vi "Get Measurement Plug-in API Paths.vi"(11 "error in":errorcluster) -> (6 "meas plugin api paths":path[](array[path]), 15 "error out":errorcluster)   [LabVIEW 2021, in "Path Functions.lvlib"]
uses:
  Path Functions.lvlib
  e97babff-5d82-41c0-a956-71097acbec5b.vi
  Converter Reusables/Converter Reusables.lvlib
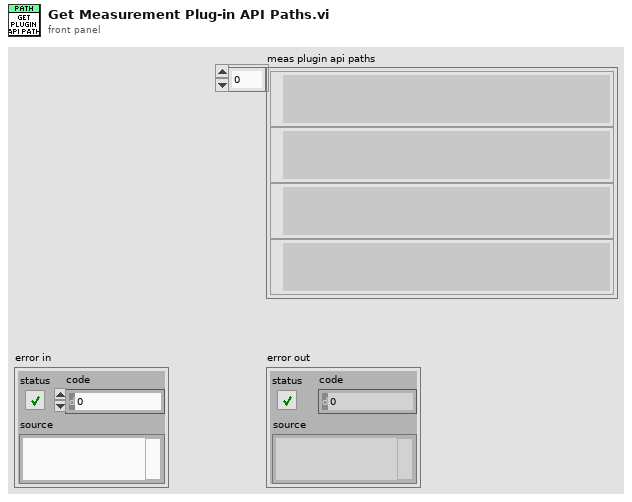
[diagram p1: front panel]
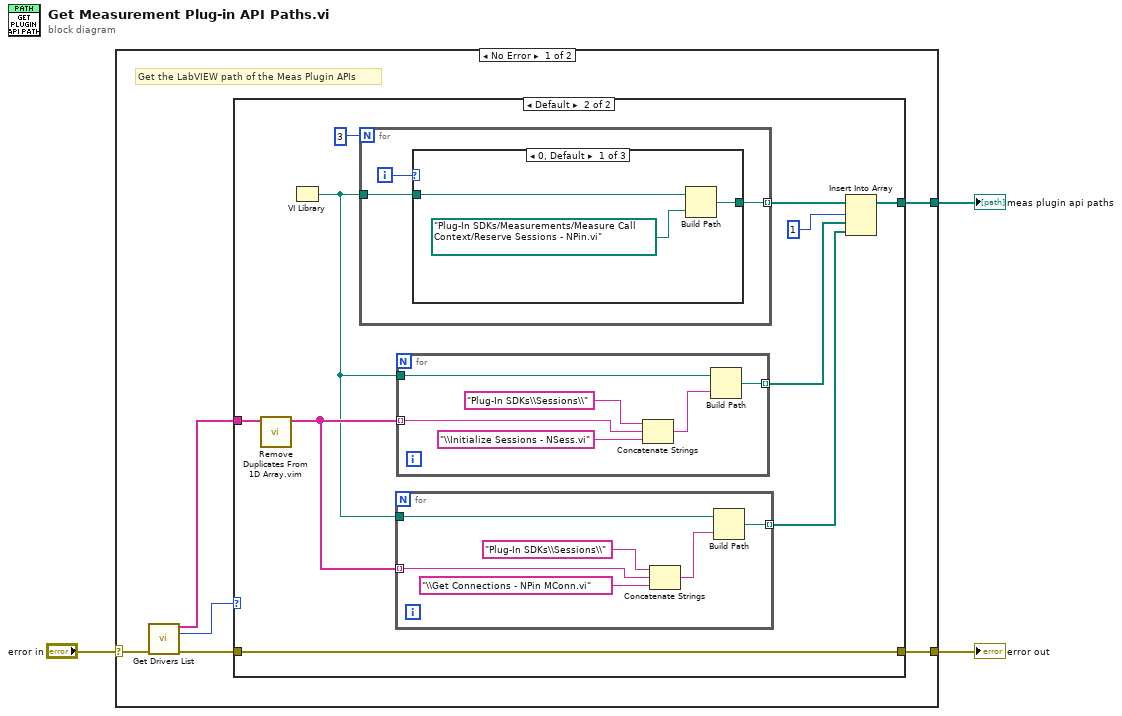
[diagram p0: block diagram]
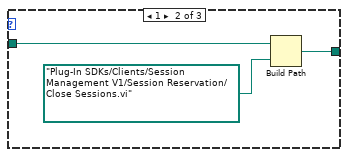
[diagram p3: hidden frame]
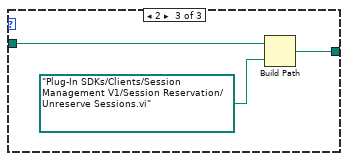
[diagram p4: hidden frame]
diagram:
  n1 = case shown="No Error" "error in" {
    selector: "error in" -> [w8 w45]
    tunnel: [w5 w45] -> w1
    tunnel: [w4 _] -> w2
    frame No Error {
      # "Get the LabVIEW path of the Meas Plugin APIs"
      n2 = call "Get Drivers List.vi"("error in"=w8) -> ("drivers list out"=w7:string[], "total driver list"=w9:i32, "error out"=w6:errorcluster)  [unwired: 9 in, 3 out]
      n3 = case shown="Default" w9 {
        tunnel: w7 -> [_ w12]
        tunnel: [w10 w13] -> w5
        tunnel: w6 -> [w10 w13]
        tunnel: [_ w11] -> w4
        frame 0 {
        }
        frame Default {
          n4 = call "Remove Duplicates From 1D Array.vim"("array"=w12) -> ("array with duplicates removed"=w19:string[])  [unwired: 10 in]
          n5 = VI Library() -> (path=w18:path)
          n6 = for {
            N: 3 -> [_]
            tunnel: w18 -> [w34]
            tunnel: [w33] -> w17 mode=indexing
            i -> [w35]
            n7 = case shown="0, Default" w35 {
              tunnel: w34 -> [w38 w40 w43]
              tunnel: [w37 w41 w44] -> w33
              frame 0, Default {
                n8 = Build Path(base path=w38, name or relative path=path "Plug-In SDKs/Measurements/Measure Call Context/Reserve Sessions - NPin.vi") -> (appended path=w37:path)
              }
              frame 1 {
                n9 = Build Path(base path=w40, name or relative path=path "Plug-In SDKs/Clients/Session Management V1/Session Reservation/Close Sessions.vi") -> (appended path=w41:path)
              }
              frame 2 {
                n10 = Build Path(base path=w43, name or relative path=path "Plug-In SDKs/Clients/Session Management V1/Session Reservation/Unreserve Sessions.vi") -> (appended path=w44:path)
              }
            }
          }
          n11 = for {
            tunnel: w18 -> [w26]
            tunnel: [w21] -> w15 mode=indexing
            tunnel: w19 -> [w25] mode=indexing
            n12 = Concatenate Strings("Plug-In SDKs\\Sessions\\" ("string"), w25, "\\Get Connections - NPin MConn.vi" ("string")) -> (w22:string)
            n13 = Build Path(base path=w26, name or relative path=w22) -> (appended path=w21:path)
          }
          n14 = for {
            tunnel: w19 -> [w29] mode=indexing
            tunnel: w18 -> [w32]
            tunnel: [w31] -> w16 mode=indexing
            n15 = Concatenate Strings("Plug-In SDKs\\Sessions\\" ("string"), w29, "\\Initialize Sessions - NSess.vi" ("string")) -> (w27:string)
            n16 = Build Path(base path=w32, name or relative path=w27) -> (appended path=w31:path)
          }
          n17 = Insert Into Array(array=w17, index=1, new element #1=w16, new element #2=w15) -> (w11:path[])
        }
      }
    }
    frame Error {
    }
  }
  "meas plugin api paths" <- w2
  "error out" <- w1
